vi "Generate and Acquire Waveform.vi"() -> ()   [LabVIEW 2010]
doc: "This example shows how to acquire 16k samples of continuous signal on fast analog inputs. Signal will be acquired simultaneously with generated signal. Time length of the acquired signal depends on the time scale of a buffer that can be set with a decimation factor. Decimations and time scales of a buffer are given in the table below. Voltage range of fast analog inputs on the Red Pitaya depends on gain setting that can be set by jumpers. HV setting is for input range to ±20V, while LV sets input range to ±1V."
uses:
  RedPitaya.lvlib
panel:
  in  "Trigger Mode":T1(ring)=enum."Ch1 positive edge"
  in  "Trigger Level (0 V)":dbl=1.1 min=-20.0 max=20.1
  in  "Delay (# Samples)":i32
  in  "Averaging":enum16{"None", "AVG ON", "AVG OFF"}(ring)
  in  "Duty Cycle":i32=-1 min=-1 max=100
  in  "Phase":i32=361
  in  "DC Offset":dbl=2.0
  in  "Amplitude":dbl=2.0
  in  "Decimation":u32(ring)=8 items=["65536"=65536, "8192"=8192, "1024"=1024, "64"=64, "8"=8, "1"=1]
  in  "Channel (1|2)":u16(ring)=1 items=["Channel 1"=1, "Channel 2"=2]
  in  "Waveform Function":u16(ring)=1 items=["", "Sine", "Square", "Triangle", "Sawtooth UP", "Sawtooth Down", "PWM"]
  in  "Frequency (1000 Hz)":i32=10000
  out "Waveform Graph":dbl[](graph)
  in  "IP address":string="192.168.1.100"
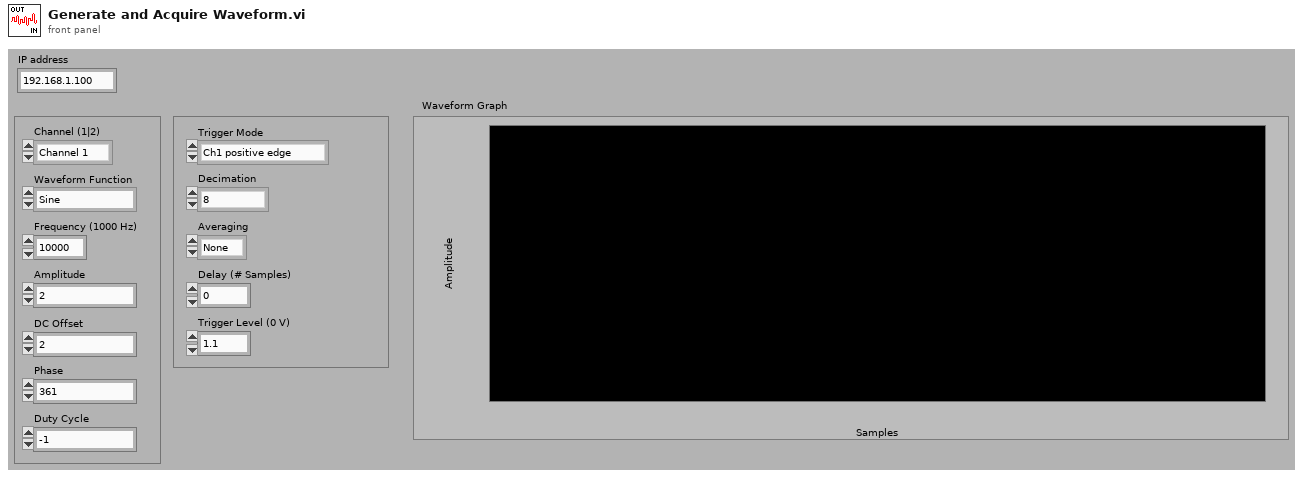
[diagram p1: front panel]
types:
  T1 = enum16{"Disabled", "Now", "Ch1 positive edge", "Ch1 negative edge", "Ch2 positive edge", "Ch2 negative edge", "external positive ege", "external negative edge", "AWG positive edge", "AWG negative edge"}
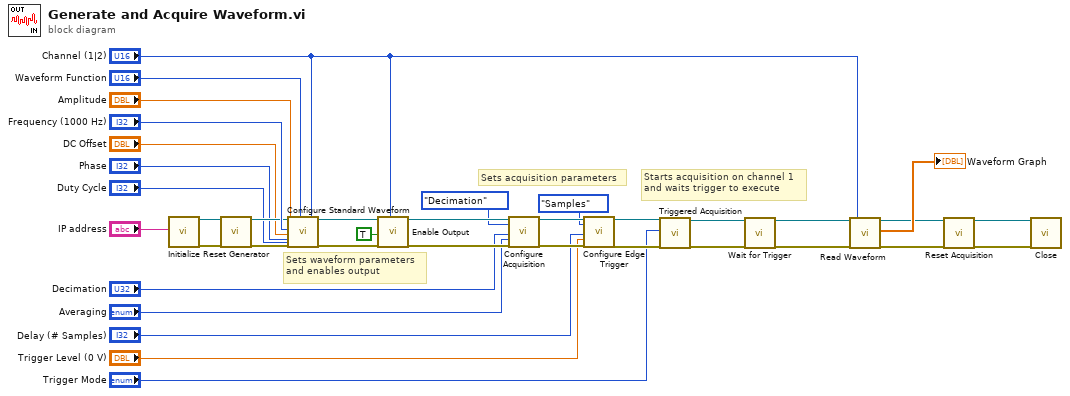
[diagram p0: block diagram]
diagram:
  # "Starts acquisition on channel 1\nand waits trigger to execute"
  # "Sets acquisition parameters"
  # "Sets waveform parameters\nand enables output"
  n1 = call "Initialize.vi"("IP address"="IP address") -> ("RedPitaya connection out"=w14:refnum<k5>, "error out"=w12:errorcluster)  [unwired: 17 in]
  n2 = call "Reset Generator.vi"("RedPitaya connection in"=w14, "error in"=w12) -> ("RedPitaya connection out"=w13:refnum<k5>, "error out"=w11:errorcluster)  [unwired: 16 in]
  n3 = call "Configure Standard Waveform.vi"("RedPitaya connection in"=w13, "Amplitude (V)"="Amplitude", "Frequency"="Frequency (1000 Hz)", "DC Offset"="DC Offset", "Phase"="Phase", "error in"=w11, "Channel #"="Channel (1|2)", "Duty Cycle"="Duty Cycle", "Waveform Function"="Waveform Function") -> ("RedPitaya connection out"=w33:refnum<k5>, "error out"=w32:errorcluster)  [unwired: 9 in]
  n4 = call "Enable Output.vi"("RedPitaya connection in"=w33, "Generation (T: Enable)"=TRUE, "error in"=w32, "Channel #"="Channel (1|2)") -> ("RedPitaya connection out"=w30:refnum<k5>, "error out"=w29:errorcluster)  [unwired: 14 in]
  n5 = call "Configure Acquisition.vi"("RedPitaya connection in"=w30, "Decimation/Sampling Rate"=enum16{"", "Sampling rate", "Decimation"}."Decimation", "Decimation"="Decimation", "Averaging"="Averaging", "error in"=w29) -> ("RedPitaya connection out"=w28:refnum<k5>, "error out"=w27:errorcluster)  [unwired: 13 in]
  n6 = call "Configure Edge Trigger.vi"("RedPitaya connection in"=w28, "Trigger Delay mode"=enum16{"", "Samples", "Nanoseconds"}."Samples", "Delay (# Samples)"="Delay (# Samples)", "Trigger Level (0 V)"="Trigger Level (0 V)", "error in"=w27) -> ("RedPitaya connection out"=w36:refnum<k5>, "error out"=w35:errorcluster)  [unwired: 13 in]
  n7 = call "Triggered Acquisition.vi"("RedPitaya TCP connection in"=w36, "Trigger Mode"="Trigger Mode", "error in"=w35) -> ("RedPitaya TCP connection out"=w26:refnum<k5>, "error out"=w23:errorcluster)  [unwired: 15 in]
  n8 = call "Wait for Trigger.vi"("RedPitaya TCP connection in"=w26, "error in"=w23) -> ("RedPitaya TCP connection out"=w25:refnum<k5>, "error out"=w24:errorcluster)  [unwired: 16 in]
  n9 = call "Read Waveform.vi"("RedPitaya TCP Connection in"=w25, "error in"=w24, "Channel #"="Channel (1|2)") -> ("RedPitaya TCP Connection out"=w22:refnum<k5>, "Measurement Array"=→"Waveform Graph":dbl[], "error out"=w20:errorcluster)  [unwired: 14 in]
  n10 = call "Reset Acquisition.vi"("RedPitaya connection in"=w22, "error in"=w20) -> ("RedPitaya connection out"=w21:refnum<k5>, "error out"=w19:errorcluster)  [unwired: 16 in]
  n11 = call "Close.vi"("RedPitaya connection in"=w21, "error in"=w19) -> ()  [unwired: 17 in, 1 out]
